vi "5492_WPI_RobotDriveRegisterEachMotor.vi"(8 "error in (no error)":errorcluster, 10 "RobotDrive refnum name":string="My RobotDrive RefNum", 11 "RobotDriveDevRef":T1={"DevStatus"={"status"=FALSE, "code"=0, "source"=""}, "Motors[]"=[], "Square Inputs"=FALSE, "Max Output"=1.0}) -> (0 "error out":errorcluster, 3 "RobotDriveDevRef Out":T1={"DevStatus"={"status"=FALSE, "code"=0, "source"=""}, "Motors[]"=[], "Square Inputs"=FALSE, "Max Output"=1.0})   [LabVIEW 2016]
uses:
  <vilib>/Rock Robotics/WPI/RobotDrive/WPI_RobotDriveDevRef.ctl
  <vilib>/Rock Robotics/WPI/MotorControl/WPI_MotorControlDeviceRef.ctl
  <vilib>/Rock Robotics/WPI/MotorControl/WPI_MotorControlType.ctl
  <vilib>/Rock Robotics/SystemInterfaces/DIO/FPGA_DIOPWMChannel.ctl
  <vilib>/Rock Robotics/WPI/PWM/WPI_PWMDeadband.ctl
  5492_WPI_RobotDriveMotorSelectorEnum.ctl
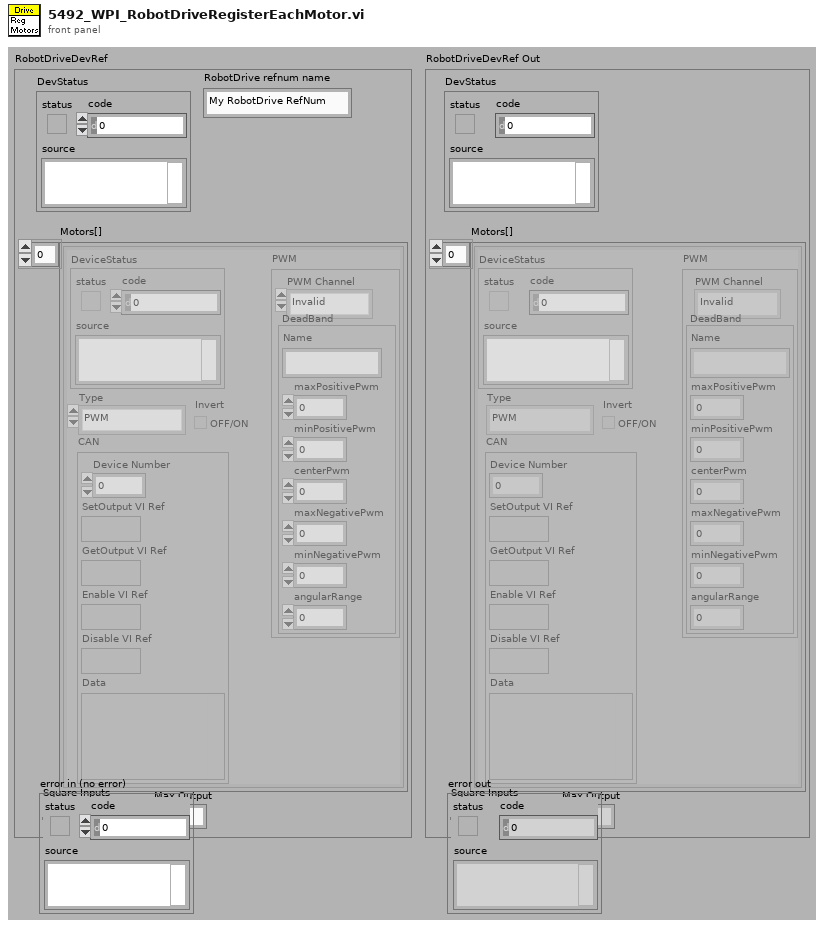
[diagram p1: front panel]
types:
  T1 = typedef "WPI_RobotDriveDevRef.ctl" = cluster{"DevStatus":errorcluster, "Motors[]":T2[], "Square Inputs":bool, "Max Output":dbl}
  T2 = typedef "WPI_MotorControlDeviceRef.ctl" = cluster{"DeviceStatus":errorcluster, "Type":T3, "PWM":cluster{"PWM Channel":T4, "DeadBand":T5}, "CAN":cluster{"Device Number":u8, "SetOutput VI Ref":variant, "GetOutput VI Ref":variant, "Enable VI Ref":variant, "Disable VI Ref":variant, "Data":variant}, "Invert":bool}
  T3 = typedef "WPI_MotorControlType.ctl" = enum16{"PWM", "CAN"}
  T4 = typedef "FPGA_DIOPWMChannel.ctl" = enum8{"PWM 0", "PWM 1", "PWM 2", "PWM 3", "PWM 4", "PWM 5", "PWM 6", "PWM 7", "PWM 8", "PWM 9", "PWM MXP 0", "PWM MXP 1", "PWM MXP 2", "PWM MXP 3", "PWM MXP 4", "PWM MXP 5", "PWM MXP 6", "PWM MXP 7", "PWM MXP 8", "PWM MXP 9", "Invalid"}
  T5 = typedef "WPI_PWMDeadband.ctl" = cluster{"Name":string, "maxPositivePwm":i32, "minPositivePwm":i32, "centerPwm":i32, "maxNegativePwm":i32, "minNegativePwm":i32, "angularRange":u16}
  T6 = typedef "5492_WPI_RobotDriveMotorSelectorEnum.ctl" = enum16{"Front left motor", "Front right motor", "Back left motor", "Back right motor", "Middle left motor", "Middle right motor"}
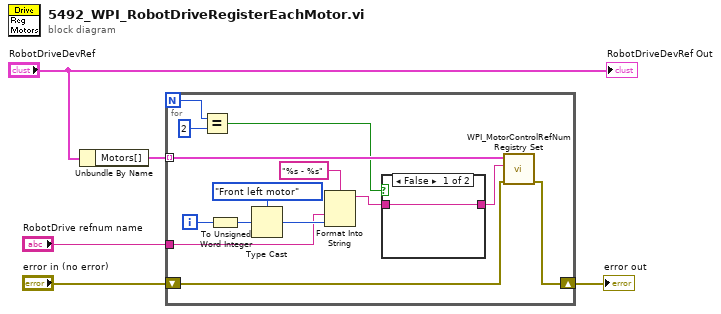
[diagram p0: block diagram]
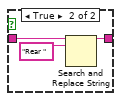
[diagram p2: hidden frame]
diagram:
  n1 = Unbundle By Name("RobotDriveDevRef") -> ("Motors[]"=w5:T2[])
  n2 = for {
    N -> [w17]
    tunnel: w5 -> [w14] mode=indexing
    tunnel: "RobotDrive refnum name" -> [w10]
    shift-right: [w8] -> w1
    shift-left: "error in (no error)" -> [w9]
    i -> [w7]
    n3 = Equal?(x=w17, y=2) -> (x = y?=w12:bool)
    n4 = To Unsigned Word Integer(number=w7) -> (unsigned 16bit integer=w6:u16)
    n5 = Type Cast(type=5492_WPI_RobotDriveMotorSelectorEnum."Front left motor" ("Motor Selector Enum"), x=w6) -> (*(type *) &x=w15:T6)
    n6 = Format Into String(format string="%s - %s", w10, w15) -> (resulting string=w13:string)  [unwired: 2 in, 1 out]
    n7 = case shown="False" w12 {
      tunnel: w13 -> [w20 w23]
      tunnel: [w20 w22] -> w11
      frame False {
      }
      frame True {
        n8 = Search and Replace String(input string=w23, search string="Rear ") -> (result string=w22:string)  [unwired: 1 in, 8 out]
      }
    }
    n9 = call <vilib>:"WPI_MotorControlRefNum Registry Set.vi"("error in (no error)"=w9, "refnum name"=w11, "MotorControlDevRef"=w14) -> ("error out"=w8:errorcluster)  [unwired: 1 in, 7 out]
  }
  "error out" <- w1
  "RobotDriveDevRef Out" <- "RobotDriveDevRef"
